vi "20190110_Shift_00_ATA_FPGA.vi"(6 "Scale":T2={"Scale_Step4"=1.0, "Scale_Step5"=1.0, "Scale_Step6"=1.0, "Scale_Step7"=1.0}, 7 "Input valid":bool, 8 "EnableFIFO":bool, 9 "Enable":T3, 10 "frequency shift":fxp<+/-,48,0> format="%#.48g", 11 "Data in":fxp<+/-,18,1>) -> (0 "Q Probe":T1, 1 "Q Data out":fxp<+/-,24,1>, 2 "I Probe":T1, 3 "I Data out":fxp<+/-,24,1>, 5 "output valid":bool)   [LabVIEW 2018]
uses:
  <instrlib>/_niInstr/DSP/v1/Shared/Public/IQ Data.ctl
  <instrlib>/_niInstr/DSP/v1/Shared/niInstr DSP v1 Shared.lvlib
  FPGA_Controls/FPGA_Probe_Clust.ctl
  <instrlib>/_niInstr/DSP/v1/FPGA/niInstr DSP v1 FPGA.lvlib
  <instrlib>/_niInstr/DSP/v1/FPGA/Public/Sub VIs/Frequency Shift/Frequency Shift - 1 spc.vi
  FPGA_Controls/FPGA_Enable_Clust.ctl
  FPGA_Controls/FPGA_Scale_Clust.ctl
panel:
  out "Q Index":i32
  out "I Index":i32
  in  "Index":i32
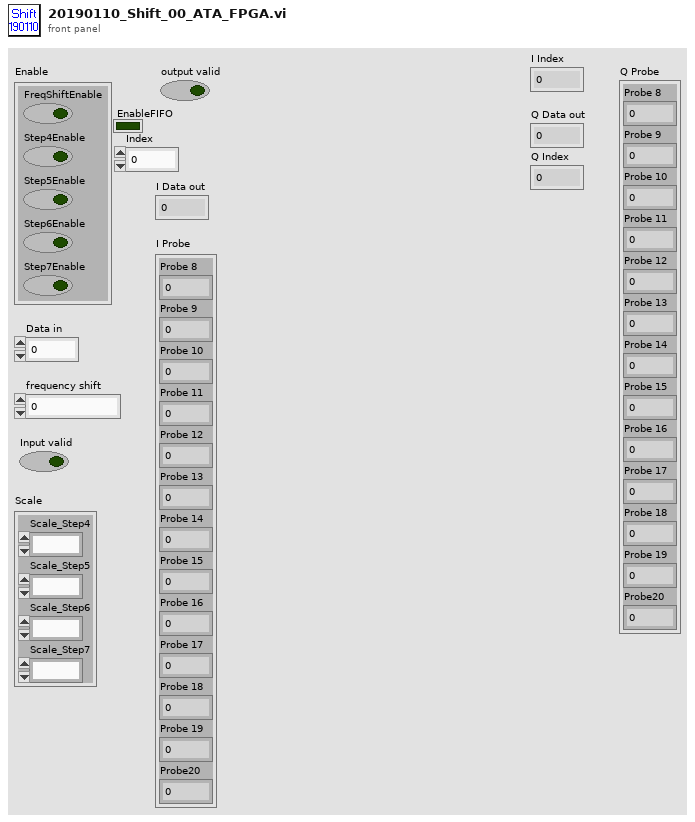
[diagram p1: front panel]
types:
  T1 = typedef "FPGA_Probe_Clust.ctl" = cluster{"Probe 8":fxp<+/-,18,1>, "Probe 9":fxp<+/-,24,1>, "Probe 10":fxp<+/-,24,1>, "Probe 11":fxp<+/-,24,1>, "Probe 12":fxp<+/-,47,24>, "Probe 13":fxp<+/-,24,1>, "Probe 14":fxp<+/-,25,2>, "Probe 15":fxp<+/-,48,25>, "Probe 16":fxp<+/-,24,1>, "Probe 17":fxp<+/-,25,2>, "Probe 18":fxp<+/-,48,25>, "Probe 19":fxp<+/-,24,1>, "Probe20":fxp<+/-,24,1>}
  T2 = typedef "FPGA_Scale_Clust.ctl" = cluster{"Scale_Step4":fxp<+/-,23,23>, "Scale_Step5":fxp<+/-,23,23>, "Scale_Step6":fxp<+/-,23,23>, "Scale_Step7":fxp<+/-,23,23>}
  T3 = typedef "FPGA_Enable_Clust.ctl" = cluster{"FreqShiftEnable":bool, "Step4Enable":bool, "Step5Enable":bool, "Step6Enable":bool, "Step7Enable":bool}
  T4 = typedef "niInstr DSP v1 Shared.lvlib/IQ Data.ctl" = cluster{"I":fxp<+/-,18,1>, "Q":fxp<+/-,18,1>, "overflow":bool}
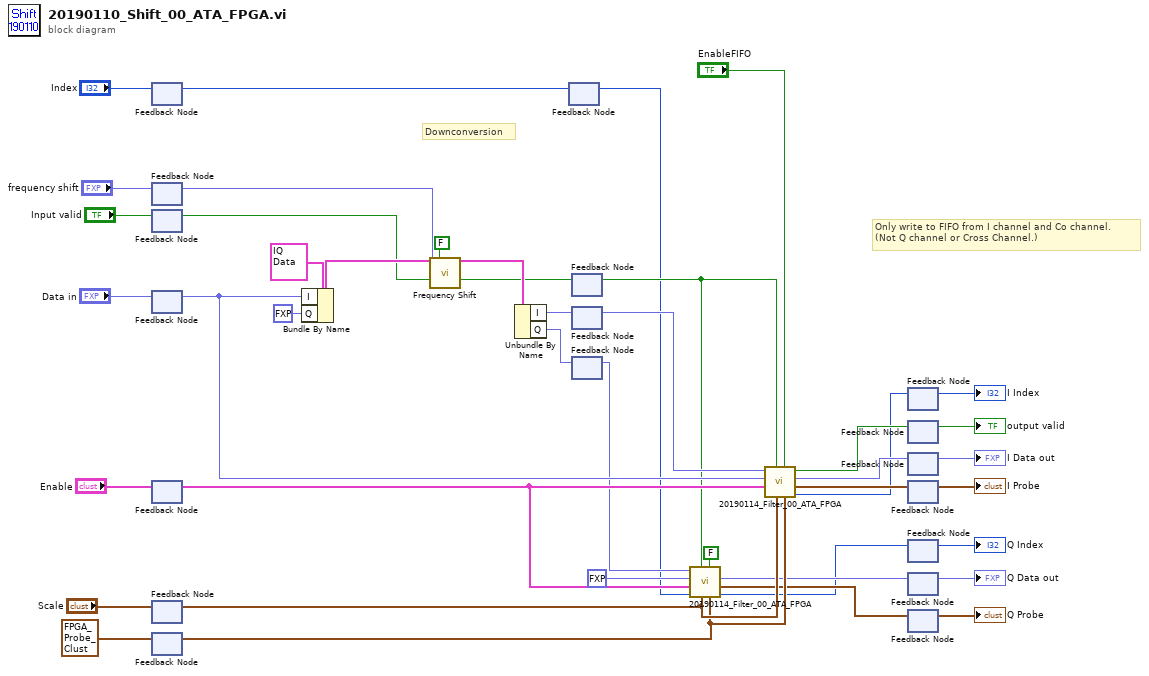
[diagram p0: block diagram]
diagram:
  # "Only write to FIFO from I channel and Co channel.\n(Not Q channel or Cross Channel.)"
  # "Downconversion"
  n1 = feedback #1() -> (w6:i32)  [unwired: 1 in]
  n2 = feedback-in #1("Index") -> ()
  n3 = feedback #2() -> (w29:fxp<+/-,48,0>)  [unwired: 1 in]
  n4 = feedback-in #2("frequency shift") -> ()
  n5 = feedback #3() -> (w31:bool)  [unwired: 1 in]
  n6 = feedback-in #3("Input valid") -> ()
  n7 = feedback #4() -> (w35:fxp<+/-,18,1>)  [unwired: 1 in]
  n8 = feedback-in #4("Data in") -> ()
  n9 = feedback #5() -> (w33:T3)  [unwired: 1 in]
  n10 = feedback-in #5("Enable") -> ()
  n11 = feedback #6() -> (w27:T2)  [unwired: 1 in]
  n12 = feedback-in #6("Scale") -> ()
  n13 = feedback #7() -> (w25:T1)  [unwired: 1 in]
  n14 = feedback-in #7(T1 {"Probe 8"=0.0, "Probe 9"=0.0, "Probe 10"=0.0, "Probe 11"=0.0, "Probe 12"=0.0, "Probe 13"=0.0, "Probe 14"=0.0, "Probe 15"=0.0, "Probe 16"=0.0, "Probe 17"=0.0, "Probe 18"=0.0, "Probe 19"=0.0, "Probe20"=0.0} ("Probe 9")) -> ()
  n15 = Bundle By Name(cluster=T4 {"I"=0.0, "Q"=0.0, "overflow"=FALSE} ("data"), "I"=w35, "Q"=fxp<+/-,18,1> 0.0) -> (w40:T4)
  n16 = call-poly <instrlib>:"Frequency Shift.vi"("data in"=w40, "reset"=FALSE, "frequency shift"=w29, "input valid"=w31) -> ("data out"=w39:T4, "output valid"=w21:bool)  [unwired: 8 in, 2 out]
  n17 = Unbundle By Name(w39) -> ("I"=w23:fxp<+/-,18,1>, "Q"=w24:fxp<+/-,18,1>)
  n18 = feedback #8() -> (w5:i32)  [unwired: 1 in]
  n19 = feedback-in #8(w6) -> ()
  n20 = feedback #9() -> (w20:bool)  [unwired: 1 in]
  n21 = feedback-in #9(w21) -> ()
  n22 = feedback #10() -> (w22:fxp<+/-,18,1>)  [unwired: 1 in]
  n23 = feedback-in #10(w23) -> ()
  n24 = feedback #11() -> ()  [unwired: 2 in]
  n25 = feedback-in #11(w24) -> ()
  n26 = call "20190114_Filter_00_ATA_FPGA.vi"("Probe 10"=w25, "EnableFIFO"=FALSE, "Scale"=w27, "output valid in"=w20, "Index"=w5, "Enable"=w33, "UnshiftedData"=fxp<+/-,18,1> 0.0, "ShiftedData"=w24) -> ("Index out"=w2:u32, "Probe 9"=w15:T1, "fixed-point type"=w16:fxp<+/-,24,1>)  [unwired: 1 out]
  n27 = call "20190114_Filter_00_ATA_FPGA.vi"("Probe 10"=w25, "EnableFIFO"="EnableFIFO", "Scale"=w27, "output valid in"=w20, "Enable"=w33, "UnshiftedData"=w35, "ShiftedData"=w22) -> ("Index out"=w4:u32, "Probe 9"=w17:T1, "fixed-point type"=w18:fxp<+/-,24,1>, "output valid out"=w19:bool)  [unwired: 1 in]
  n28 = feedback #12() -> (→"I Index":u32)  [unwired: 1 in]
  n29 = feedback-in #12(w4) -> ()
  n30 = feedback #13() -> (→"output valid":bool)  [unwired: 1 in]
  n31 = feedback-in #13(w19) -> ()
  n32 = feedback #14() -> (→"I Data out":fxp<+/-,24,1>)  [unwired: 1 in]
  n33 = feedback-in #14(w18) -> ()
  n34 = feedback #15() -> (→"I Probe":T1)  [unwired: 1 in]
  n35 = feedback-in #15(w17) -> ()
  n36 = feedback #16() -> (→"Q Index":u32)  [unwired: 1 in]
  n37 = feedback-in #16(w2) -> ()
  n38 = feedback #17() -> (→"Q Data out":fxp<+/-,24,1>)  [unwired: 1 in]
  n39 = feedback-in #17(w16) -> ()
  n40 = feedback #18() -> (→"Q Probe":T1)  [unwired: 1 in]
  n41 = feedback-in #18(w15) -> ()
